vi "STRING_POT_CAL 2016.vi"(6 "Sensor Cluster":T1, 7 "Array in":refnum<k24>[](array[refnum]), 8 "error in (no error)":errorcluster, 9 "Descriptions":string[](array[string]), 11 "string_pot_slope_IN":dbl=51.35 format="%.2f") -> (0 "error out":errorcluster, 3 "string_pot_slope_OUT":dbl=51.35 format="%.2f", 4 "Sensor Cluster 2":T1, 5 "Array out":refnum<k24>[](array[refnum]))   [LabVIEW 2016]
uses:
  C:/Program Files (x86)/National Instruments/LabVIEW 2016/vi.lib/ULx/ULx_LV.dll
  Waterloo DAQ/controls/MCC DAQ Readings.ctl
  KPRO_lv2015/ad interface/Global_SIM_switch.vi
  KPRO_lv2015/Kpro Globals.vi
panel:
  out "Distance(ft)":dbl format="%.2f"
  in  "stop":bool
  in  "start":bool
  # "STRING POTENTIOMETER CALIBRATION"
  # "Hold string pot wire at 5' above the string pot body.\nPress start."
  # "Slowly lower the string pot wire.\nPress Stop when t he string pot wire is fully retracted."
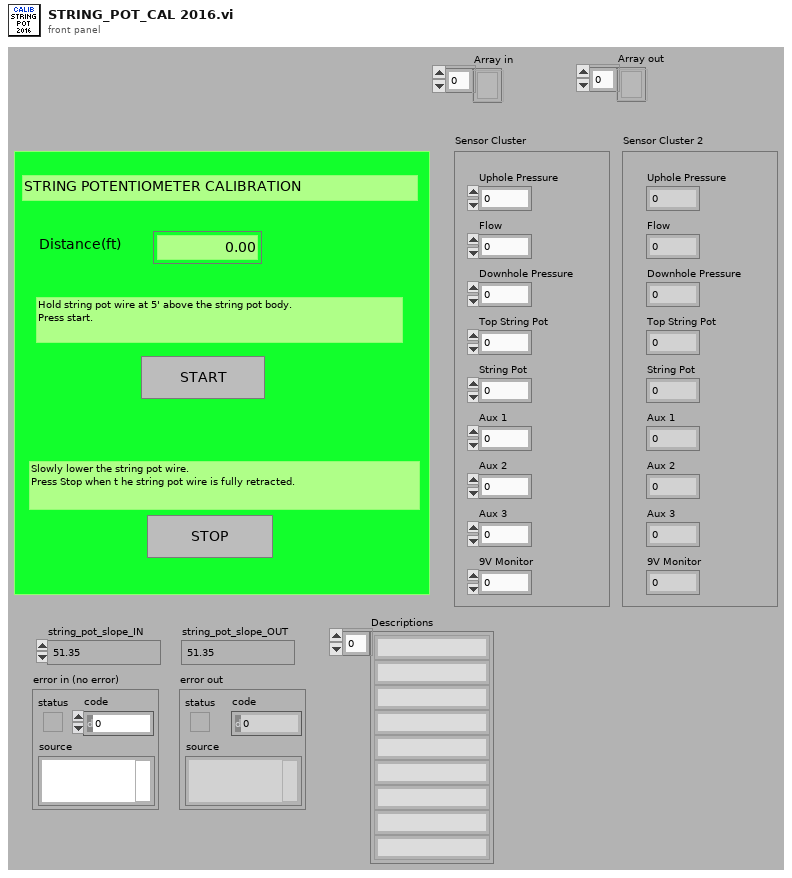
[diagram p1: front panel]
types:
  T1 = typedef "MCC DAQ Readings.ctl" = cluster{"Uphole Pressure":dbl, "Flow":dbl, "Downhole Pressure":dbl, "Top String Pot":dbl, "String Pot":dbl, "Aux 1":dbl, "Aux 2":dbl, "Aux 3":dbl, "9V Monitor":dbl}
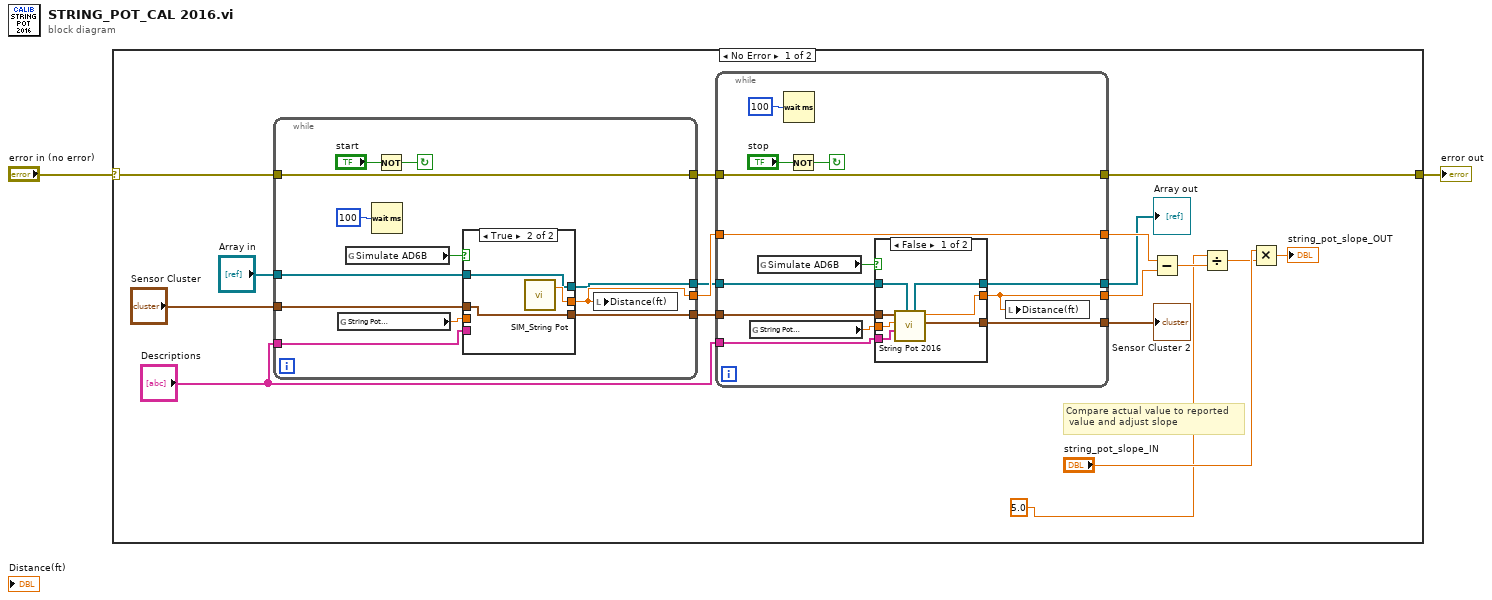
[diagram p0: block diagram]
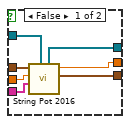
[diagram p2: hidden frame]
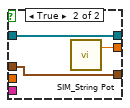
[diagram p3: hidden frame]
diagram:
  n1 = case shown="No Error" "error in (no error)" {
    selector: "error in (no error)" -> [w20 w66]
    tunnel: [w18 w66] -> w2
    frame No Error {
      # "Compare actual value to reported\n value and adjust slope"
      n2 = while {
        tunnel: [w27] -> w15
        tunnel: [w30] -> w19
        tunnel: w20 -> [w30]
        tunnel: "Array in" -> [w26]
        tunnel: "Sensor Cluster" -> [w25]
        tunnel: "Descriptions" -> [w24]
        tunnel: [w23] -> w5
        tunnel: [w22] -> w7
        stop <- w31 continue-if-true
        n3 = global read "Kpro Globals.vi" "String Pot \nSlope"() -> (w21:dbl)
        n4 = global read "Global_SIM_switch.vi" "Simulate AD6B"() -> (w29:bool)
        n5 = Wait (ms)(milliseconds to wait=u32 100) -> ()  [unwired: 1 out]
        n6 = Not(x="start") -> (.not. x?=w31:bool)
        n7 = case shown="True" w29 {
          tunnel: [w39 w42] -> w27
          tunnel: w26 -> [w38 w40]
          tunnel: w25 -> [w37 w41]
          tunnel: w24 -> [w36 _]
          tunnel: [w35 w41] -> w23
          tunnel: [w34 w40] -> w22
          tunnel: w21 -> [w33 _]
          frame False {
            n8 = call "String Pot 2016.vi"("Array in"=w38, "Descriptions"=w36, "String Pot \nSlope"=w33, "Sensor Cluster"=w37) -> ("Sensor Cluster 2"=w35:T1, "Distance (in)"=w39:dbl, "Array out"=w34:refnum<k24>[])  [unwired: 4 in, 1 out]
          }
          frame True {
            n9 = call "SIM_String Pot.vi"() -> ("Distance (in)"=w42:dbl)  [unwired: 3 in]
          }
        }
        n10 = local write "Distance(ft)"(w27) -> ()
      }
      n11 = while {
        tunnel: w15 -> [w52]
        tunnel: [w50] -> w12
        tunnel: [w52] -> w11
        tunnel: w19 -> [w53]
        tunnel: [w53] -> w18
        tunnel: "Descriptions" -> [w48]
        tunnel: w7 -> [w47]
        tunnel: [w46] -> w6
        tunnel: w5 -> [w44]
        tunnel: [w43] -> w4
        stop <- w55 continue-if-true
        n12 = global read "Kpro Globals.vi" "String Pot \nSlope"() -> (w45:dbl)
        n13 = global read "Global_SIM_switch.vi" "Simulate AD6B"() -> (w49:bool)
        n14 = Wait (ms)(milliseconds to wait=u32 100) -> ()  [unwired: 1 out]
        n15 = Not(x="stop") -> (.not. x?=w55:bool)
        n16 = case shown="False" w49 {
          tunnel: [w62 w65] -> w50
          tunnel: w47 -> [w61 w63]
          tunnel: w44 -> [w60 w64]
          tunnel: w48 -> [w59 _]
          tunnel: [w58 w64] -> w43
          tunnel: [w57 w63] -> w46
          tunnel: w45 -> [w56 _]
          frame False {
            n17 = call "String Pot 2016.vi"("Array in"=w61, "Descriptions"=w59, "String Pot \nSlope"=w56, "Sensor Cluster"=w60) -> ("Sensor Cluster 2"=w58:T1, "Distance (in)"=w62:dbl, "Array out"=w57:refnum<k24>[])  [unwired: 4 in, 1 out]
          }
          frame True {
            n18 = call "SIM_String Pot.vi"() -> ("Distance (in)"=w65:dbl)  [unwired: 3 in]
          }
        }
        n19 = local write "Distance(ft)"(w50) -> ()
      }
      "Sensor Cluster 2" <- w4
      "Array out" <- w6
      n20 = Subtract(x=w11, y=w12) -> (x-y=w14:dbl)
      n21 = Divide(x=5.0, y=w14) -> (x/y=w13:dbl)
      n22 = Multiply(x="string_pot_slope_IN", y=w13) -> (x*y=→"string_pot_slope_OUT":dbl)
    }
    frame Error {
    }
  }
  "error out" <- w2
